vi "FeedbackDecode_GenContStimFreq.vi"(3 "EncodeClust":T1={"ParamsTable"=[], "Sel"=[], "Stim"=FALSE, "StimMode"=enum."Off", "StimStep"=[enum."1uA", enum."1uA", enum."Off"], "Jitter"=FALSE, "Pulse"=FALSE, "BFreq"=0.0, "BAmp"=0.0, "UEAArray"=[], "AdjClust"={"Add"=FALSE, "Sub"=FALSE, "Val"=[1.0, 100.0, 0.2, 500.0, 0.0], "B"=[FALSE, FALSE, FALSE, FALSE, FALSE], "Inc+"=["x+1", "x+10", "x+0.1", "x+10", "x+10"], "Set"=FALSE, "LoadTable"=FALSE, "SaveTable"=FALSE, "ClearTable"=FALSE, "DeleteSel"=FALSE, "Inc-"=["x-1", "x-10", "x-0.1", "x-10", "x-10"]}, "PresetTable"=[], "SelPreset"=[], "SortClust"={"Region"=FALSE, "Receptor"=FALSE, "Electrode"=FALSE, "Min Amp"=FALSE, "Max Amp"=FALSE, "Min Freq"=FALSE, "Max Freq"=FALSE, "Duration"=FALSE}, "SelSort"={"Sel"=FALSE}, "PresetClust"={"Load"=FALSE, "Clear"=FALSE, "Save"=FALSE, "Del"=FALSE}, "RespClust"={"RespType"=enum."Sensor Map", "OpenResp"=FALSE}, "AmpLimit"=0.0, "FreqLimit"=0.0, "DurLimit"=0.0, "Wait Period"=0.0, "Train Period"=0.0, "ManualType"=enum."Max"} {"Train Period" min=0.0 max=100.0 step=0.1; "Wait Period" min=0.0 max=100.0 step=0.1; "DurLimit" min=0.0 max=1.0 step=0.01; "FreqLimit" min=0.0 max=500.0 step=1.0; "AmpLimit" min=0.0 max=100.0 step=1.0; "BAmp" min=0.0 max=100.0 step=1.0; "BFreq" min=0.0 max=100.0 step=1.0}, 4 "TargDist":dbl[](array[numeric])=[0.0, 0.0, 0.0, 0.0, 0.0, 0.0], 5 "State":T2(ring)) -> (1 "ContStimFreq":dbl[](array[numeric]))   [LabVIEW 2020]
uses:
  FeedbackDecode_EncodeClust.ctl
panel:
  # "Sends a continous frequency array to ML that corresponds to the 6 targets (thumb,index,middle,ring,little,wrist). If Mode is set to MSMS and TargDist is greater than 1 and State is AcquireResponse, ContStimFreq will be scaled from MinFreq to MaxFreq. Region must be thumb_distal, index_distal, middle_distal, ring_distal, pinky_distal, or palm_side. All other conditions result in ContStimFreq set to zero. A zero value will stop stimulation on the ML side."
  # "Value"
  # "Inc-"
  # "Inc+"
  # "Min Amp"
  # "Max Amp"
  # "Min Freq"
  # "Max Freq"
  # "Duration"
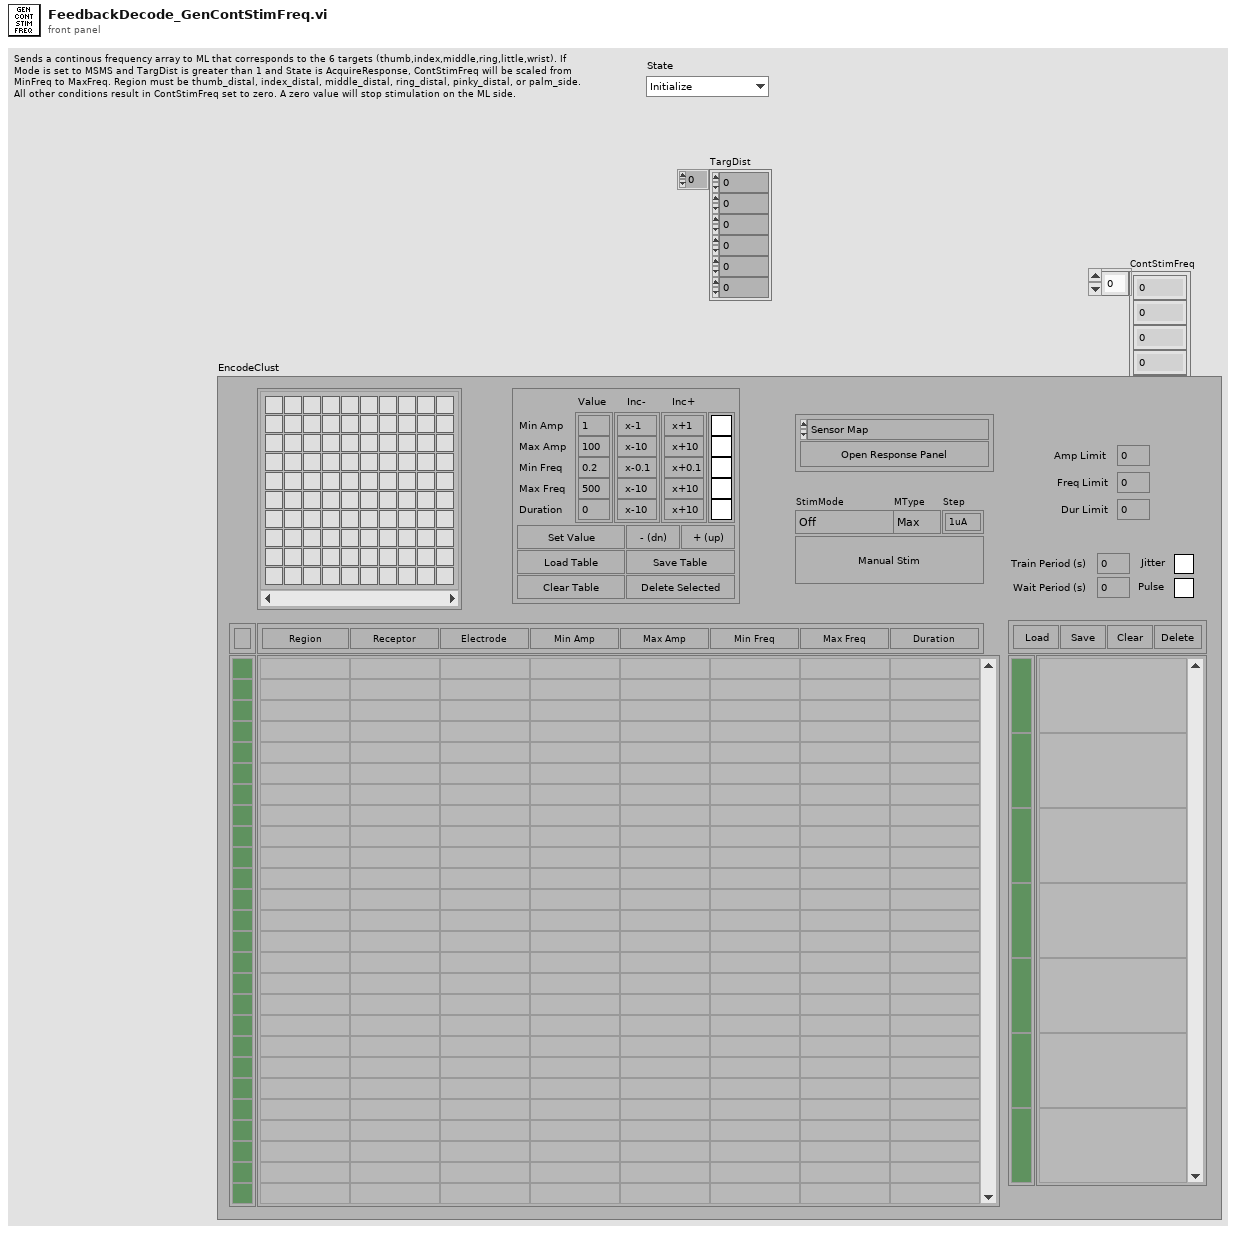
[diagram p1: front panel]
types:
  T1 = typedef "FeedbackDecode_EncodeClust.ctl" = cluster{"ParamsTable":string[][], "Sel":bool[], "Stim":bool, "StimMode":enum16{"Off", "Manual", "MSMS", "VRE", "3DHand", "DEKA", "Analog(DEKA)"}, "StimStep":enum16{"Off", "1uA", "2uA", "5uA", "10uA", "20uA", "30uA"}[], "Jitter":bool, "Pulse":bool, "BFreq":dbl, "BAmp":dbl, "UEAArray":cluster{"Boolean 1":bool, "Boolean 2":bool, "Boolean 3":bool, "Boolean 4":bool, "Boolean 5":bool, "Boolean 6":bool, "Boolean 7":bool, "Boolean 8":bool, "Boolean 9":bool, "Boolean 10":bool, "Boolean 11":bool, "Boolean 12":bool, "Boolean 13":bool, "Boolean 14":bool, "Boolean 15":bool, "Boolean 16":bool, "Boolean 17":bool, "Boolean 18":bool, "Boolean 19":bool, "Boolean 20":bool, "Boolean 21":bool, "Boolean 22":bool, "Boolean 23":bool, "Boolean 24":bool, "Boolean 25":bool, "Boolean 26":bool, "Boolean 27":bool, "Boolean 28":bool, "Boolean 29":bool, "Boolean 30":bool, "Boolean 31":bool, "Boolean 32":bool, "Boolean 33":bool, "Boolean 34":bool, "Boolean 35":bool, "Boolean 36":bool, "Boolean 37":bool, "Boolean 38":bool, "Boolean 39":bool, "Boolean 40":bool, "Boolean 41":bool, "Boolean 42":bool, "Boolean 43":bool, "Boolean 44":bool, "Boolean 45":bool, "Boolean 46":bool, "Boolean 47":bool, "Boolean 48":bool, "Boolean 49":bool, "Boolean 50":bool, "Boolean 51":bool, "Boolean 52":bool, "Boolean 53":bool, "Boolean 54":bool, "Boolean 55":bool, "Boolean 56":bool, "Boolean 57":bool, "Boolean 58":bool, "Boolean 59":bool, "Boolean 60":bool, "Boolean 61":bool, "Boolean 62":bool, "Boolean 63":bool, "Boolean 64":bool, "Boolean 65":bool, "Boolean 66":bool, "Boolean 67":bool, "Boolean 68":bool, "Boolean 69":bool, "Boolean 70":bool, "Boolean 71":bool, "Boolean 72":bool, "Boolean 73":bool, "Boolean 74":bool, "Boolean 75":bool, "Boolean 76":bool, "Boolean 77":bool, "Boolean 78":bool, "Boolean 79":bool, "Boolean 80":bool, "Boolean 81":bool, "Boolean 82":bool, "Boolean 83":bool, "Boolean 84":bool, "Boolean 85":bool, "Boolean 86":bool, "Boolean 87":bool, "Boolean 88":bool, "Boolean 89":bool, "Boolean 90":bool, "Boolean 91":bool, "Boolean 92":bool, "Boolean 93":bool, "Boolean 94":bool, "Boolean 95":bool, "Boolean 96":bool, "Boolean 97":bool, "Boolean 98":bool, "Boolean 99":bool, "Boolean 100":bool}[], "AdjClust":cluster{"Add":bool, "Sub":bool, "Val":dbl[], "B":bool[], "Inc+":string[], "Set":bool, "LoadTable":bool, "SaveTable":bool, "ClearTable":bool, "DeleteSel":bool, "Inc-":string[]}, "PresetTable":string[][], "SelPreset":bool[], "SortClust":cluster{"Region":bool, "Receptor":bool, "Electrode":bool, "Min Amp":bool, "Max Amp":bool, "Min Freq":bool, "Max Freq":bool, "Duration":bool}, "SelSort":cluster{"Sel":bool}, "PresetClust":cluster{"Load":bool, "Clear":bool, "Save":bool, "Del":bool}, "RespClust":cluster{"RespType":enum16{"Sensor Map", "Full Map"}, "OpenResp":bool}, "AmpLimit":dbl, "FreqLimit":dbl, "DurLimit":dbl, "Wait Period":dbl, "Train Period":dbl, "ManualType":enum16{"Max", "Min"}}
  T2 = enum16{"Initialize", "Acquire Start", "Acquire Response", "Finalize"}
  T3 = enum16{"Off", "Manual", "MSMS", "VRE", "3DHand", "DEKA", "Analog(DEKA)"}
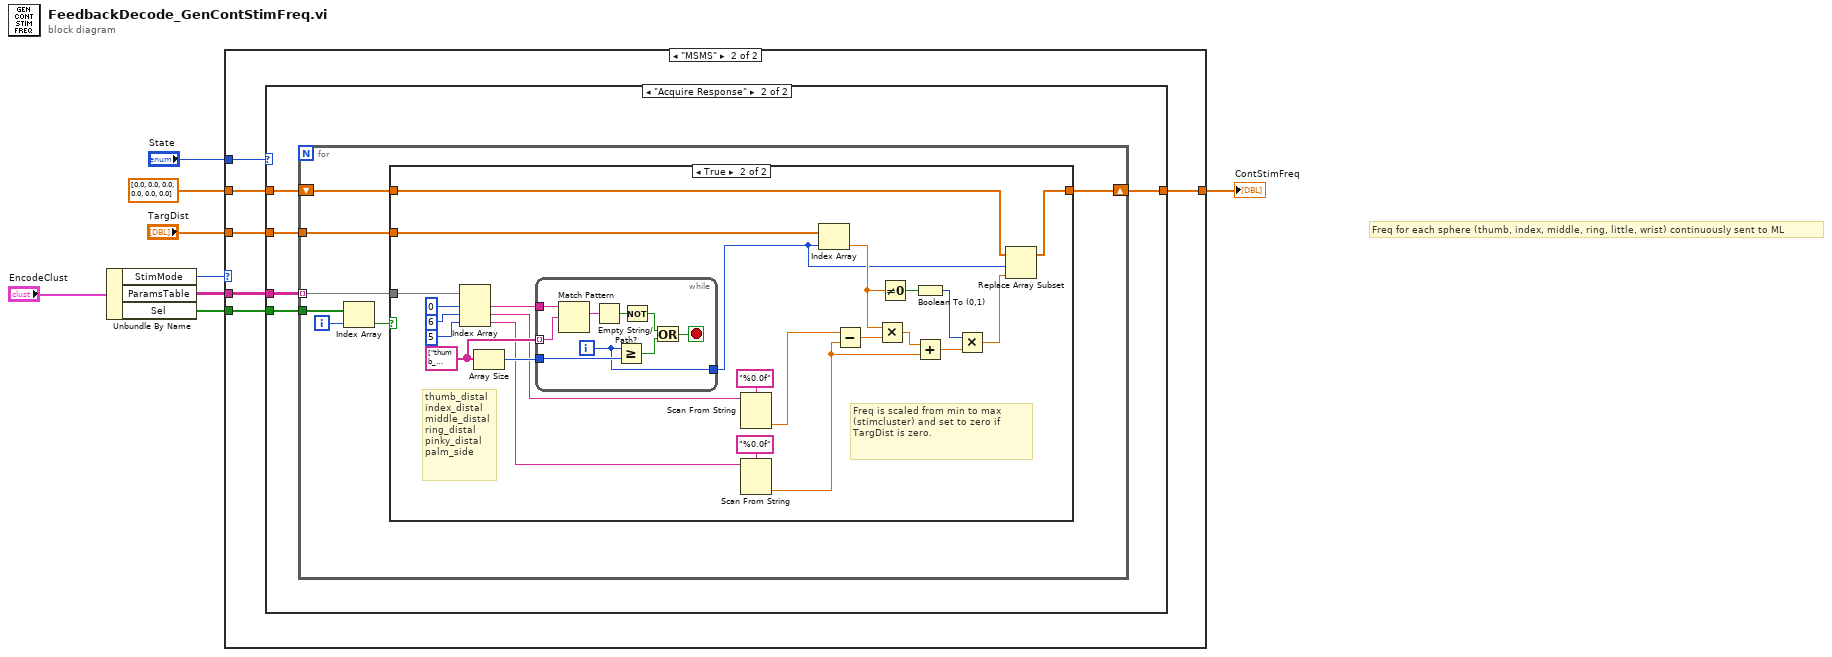
[diagram p0: block diagram]
diagram:
  # "Freq for each sphere (thumb, index, middle, ring, little, wrist) continuously sent to ML"
  n1 = Unbundle By Name("EncodeClust") -> ("StimMode"=w8:T3, "ParamsTable"=w5:string[][], "Sel"=w1:bool[])
  n2 = case shown="\"MSMS\"" w8 {
    tunnel: [w9 w11] -> w7
    tunnel: "State" -> [_ w15]
    tunnel: w5 -> [_ w14]
    tunnel: "TargDist" -> [_ w13]
    tunnel: dbl[] [0.0, 0.0, 0.0, 0.0, 0.0, 0.0] -> [w9 w12]
    tunnel: w1 -> [_ w10]
    frame "Off", Default {
    }
    frame "MSMS" {
      n3 = case shown="\"Acquire Response\"" w15 {
        tunnel: w14 -> [_ w18]
        tunnel: w13 -> [_ w21]
        tunnel: w12 -> [w16 w20]
        tunnel: [w16 w19] -> w11
        tunnel: w10 -> [_ w17]
        frame "Initialize", Default {
        }
        frame "Acquire Response" {
          n4 = for {
            tunnel: w21 -> [w28]
            shift-right: [w26] -> w19
            shift-left: w20 -> [w27]
            tunnel: w18 -> [w25] mode=indexing
            tunnel: w17 -> [w24]
            i -> [w23]
            n5 = Index Array(array=w24, index=w23) -> (element=w22:bool)
            n6 = case shown="True" w22 {
              tunnel: w28 -> [_ w53]
              tunnel: w27 -> [w29 w45]
              tunnel: [w29 w44] -> w26
              tunnel: w25 -> [_ w43]
              frame False {
              }
              frame True {
                w41 = string[] ["thumb_distal", "index_distal", "middle_distal", "ring_distal", "pinky_distal", "palm_side"]
                # "thumb_distal\nindex_distal\nmiddle_distal\nring_distal\npinky_distal\npalm_side"
                # "Freq is scaled from min to max (stimcluster) and set to zero if TargDist is zero."
                n7 = Index Array(array=w43, index #1=0 ("index"), index #2=6 ("index"), index #3=5 ("index")) -> (element #1=w42:string, element #2=w35:string, element #3=w32:string)
                n8 = Array Size(array=w41) -> (size(s)=w40:i32)
                n9 = while {
                  tunnel: w42 -> [w62]
                  tunnel: w41 -> [w61] mode=indexing
                  tunnel: w40 -> [w55]
                  tunnel: [w54] -> w39
                  i -> [w54]
                  stop <- w58 stop-if-true
                  n10 = Match Pattern(string=w62, regular expression=w61) -> (match substring=w59:string)  [unwired: 1 in, 3 out]
                  n11 = Empty String/Path?(string/path=w59) -> (empty?=w60:bool)
                  n12 = Greater Or Equal?(x=w54, y=w55) -> (x >= y?=w56:bool)
                  n13 = Not(x=w60) -> (.not. x?=w57:bool)
                  n14 = Or(x=w57, y=w56) -> (x .or. y?=w58:bool)
                }
                n15 = Scan From String(format string="%0.0f", input string=w35) -> (output 1=w31:dbl)  [unwired: 3 in, 3 out]
                n16 = Scan From String(format string="%0.0f", input string=w32) -> (output 1=w30:dbl)  [unwired: 3 in, 3 out]
                n17 = Index Array(array=w53, index=w39) -> (element=w48:dbl)
                n18 = Subtract(x=w31, y=w30) -> (x-y=w52:dbl)
                n19 = Multiply(x=w48, y=w52) -> (x*y=w51:dbl)
                n20 = Not Equal To 0?(x=w48) -> (x != 0?=w49:bool)
                n21 = Boolean To (0,1)(Boolean=w49) -> (0, 1=w47:i16)
                n22 = Add(x=w51, y=w30) -> (x+y=w50:dbl)
                n23 = Multiply(x=w47, y=w50) -> (x*y=w46:dbl)
                n24 = Replace Array Subset(array=w45, new element=w46, index=w39) -> (w44:dbl[])
              }
            }
          }
        }
      }
    }
  }
  "ContStimFreq" <- w7
